vi "SubVi Farenhait.vi"(11 "Thermometer":dbl) -> (3 "Numeric":dbl)   [LabVIEW 2020]
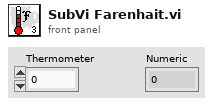
[diagram p1: front panel]
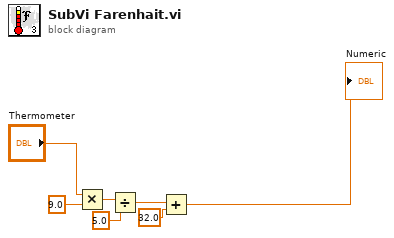
[diagram p0: block diagram]
diagram:
  n1 = Multiply(x="Thermometer", y=9.0) -> (x*y=w2:dbl)
  n2 = Divide(x=w2, y=5.0) -> (x/y=w4:dbl)
  n3 = Add(x=w4, y=32.0) -> (x+y=→"Numeric":dbl)
